vi "Voltage_Transformation[Conflict].vi"(9 "Enum":enum16{"VLN to VLL", "VLL to VLN"}(ring), 10 "Vin":sgl[](array[numeric]) format="%#_13g") -> (2 "Vout":sgl[](array[numeric]))   [LabVIEW 2018]
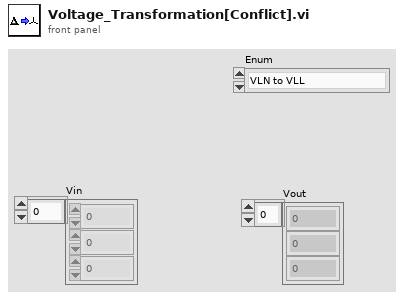
[diagram p1: front panel]
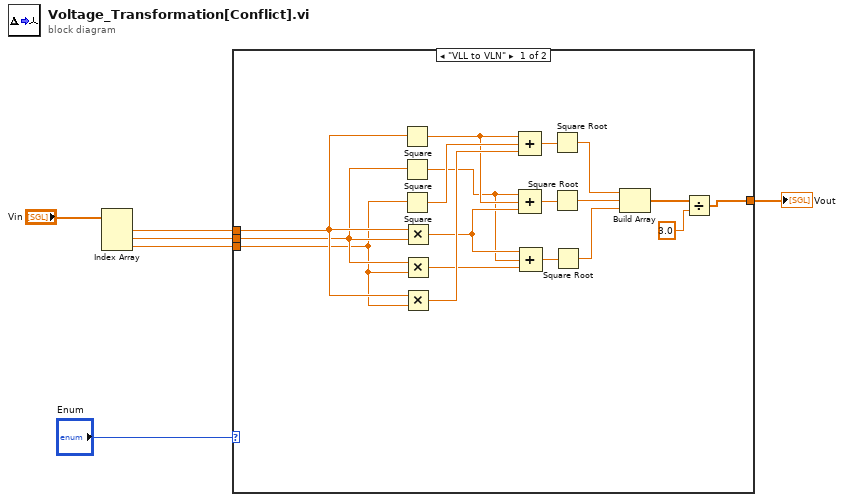
[diagram p0: block diagram]
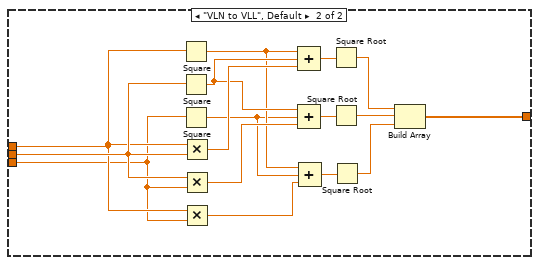
[diagram p2: hidden frame]
diagram:
  n1 = Index Array(array="Vin") -> (element #1=w4:sgl, element #2=w5:sgl, element #3=w3:sgl)  [unwired: 3 in]
  n2 = case shown="\"VLL to VLN\"" "Enum" {
    tunnel: w5 -> [w17 w40]
    tunnel: w4 -> [w18 w39]
    tunnel: w3 -> [w16 w38]
    tunnel: [w14 w31] -> w2
    frame "VLL to VLN" {
      n3 = Square(x=w18) -> (x^2=w10:sgl)
      n4 = Square(x=w17) -> (x^2=w8:sgl)
      n5 = Square(x=w16) -> (x^2=w12:sgl)
      n6 = Multiply(x=w18, y=w17) -> (x*y=w9:sgl)
      n7 = Multiply(x=w17, y=w16) -> (x*y=w7:sgl)
      n8 = Multiply(x=w18, y=w16) -> (x*y=w11:sgl)
      n9 = Compound Arithmetic op=ADD(w10, w12, w11) -> (w24:sgl)
      n10 = Compound Arithmetic op=ADD(w8, w10, w9) -> (w23:sgl)
      n11 = Compound Arithmetic op=ADD(w9, w8, w7) -> (w22:sgl)
      n12 = Square Root(x=w24) -> (sqrt(x)=w21:sgl)
      n13 = Square Root(x=w23) -> (sqrt(x)=w20:sgl)
      n14 = Square Root(x=w22) -> (sqrt(x)=w19:sgl)
      n15 = Build Array(w21, w20, w19) -> (w15:sgl[])
      n16 = Divide(x=w15, y=sgl 3.0) -> (x/y=w14:sgl[])
    }
    frame "VLN to VLL", Default {
      n17 = Square(x=w39) -> (x^2=w27:sgl)
      n18 = Square(x=w40) -> (x^2=w29:sgl)
      n19 = Square(x=w38) -> (x^2=w26:sgl)
      n20 = Multiply(x=w39, y=w40) -> (x*y=w30:sgl)
      n21 = Multiply(x=w40, y=w38) -> (x*y=w28:sgl)
      n22 = Multiply(x=w39, y=w38) -> (x*y=w25:sgl)
      n23 = Compound Arithmetic op=ADD(w27, w29, w30) -> (w37:sgl)
      n24 = Compound Arithmetic op=ADD(w29, w26, w28) -> (w36:sgl)
      n25 = Compound Arithmetic op=ADD(w27, w26, w25) -> (w35:sgl)
      n26 = Square Root(x=w37) -> (sqrt(x)=w34:sgl)
      n27 = Square Root(x=w36) -> (sqrt(x)=w33:sgl)
      n28 = Square Root(x=w35) -> (sqrt(x)=w32:sgl)
      n29 = Build Array(w34, w33, w32) -> (w31:sgl[])
    }
  }
  "Vout" <- w2
